vi "Imprimante sélection_bdd.vi"(2 "entrée d'erreur":errorcluster, 3 "Choix imprimante":string) -> (0 "sortie d'erreur":errorcluster, 1 "Output ressource VISA":refnum<visa-resource-name>="none")   [LabVIEW 2020]
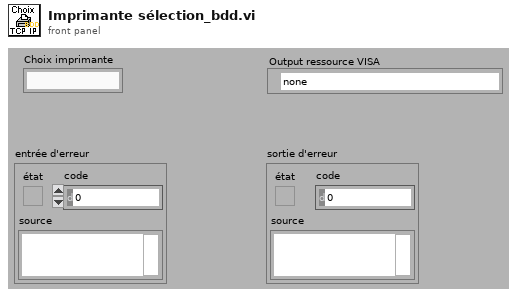
[diagram p1: front panel]
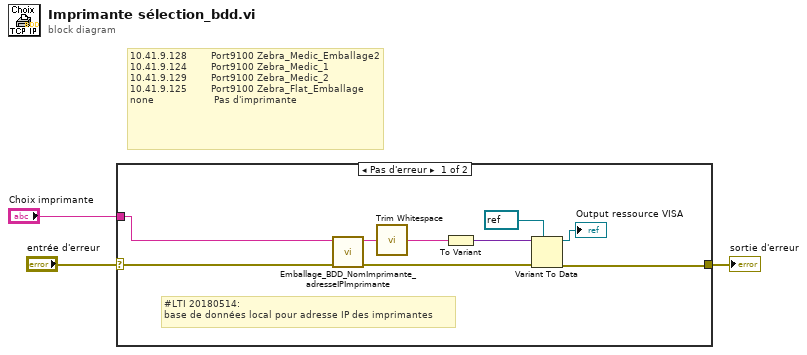
[diagram p0: block diagram]
diagram:
  # "10.41.9.128\t       Port9100\tZebra_Medic_Emballage2\n10.41.9.124       \tPort9100\tZebra_Medic_1    \n10.41.9.129\t       Port9100\tZebra_Medic_2\n10.41.9.125       \tPort9100\tZebra_Flat_Emballage\nnone                    Pas d'imprimante"
  n1 = case shown="Pas d'erreur" "entrée d'erreur" {
    selector: "entrée d'erreur" -> [w10 w13]
    tunnel: [w6 w13] -> w3
    tunnel: "Choix imprimante" -> [w5 _]
    frame No Error {
      # "#LTI 20180514:\nbase de données local pour adresse IP des imprimantes"
      n2 = call "Emballage_BDD_NomImprimante_adresseIPImprimante.vi"("Error in"=w10, "nom_imprimante"=w5) -> ("Error out"=w9:errorcluster, "élément"=w4:string)  [unwired: 8 in]
      n3 = call <vilib>:"Trim Whitespace.vi"("string"=w4) -> ("trimmed string"=w8:string)  [unwired: 1 in]
      n4 = To Variant(anything=w8) -> (Variant=w12:variant)
      n5 = Variant To Data(error in=w9, type=refnum<visa-resource-name> refnum ("Nom de ressource VISA en sortie"), Variant=w12) -> (data=→"Output ressource VISA":refnum<visa-resource-name>, error out=w6:errorcluster)
    }
    frame Error {
    }
  }
  "sortie d'erreur" <- w3
